vi "Init_Image_Dsts.vi"() -> (2 "Image Dsts Out":T2)   [LabVIEW 2011]
uses:
  <vilib>/vision/Image Controls.llb/IMAQ Image.ctl
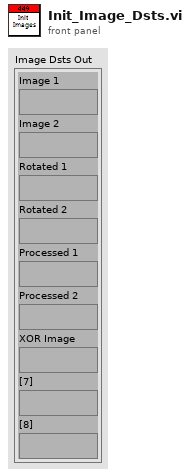
[diagram p1: front panel]
types:
  T1 = typedef "IMAQ Image.ctl" = refnum<image>
  T2 = cluster{"Image 1":T1, "Image 2":T1, "Rotated 1":T1, "Rotated 2":T1, "Processed 1":T1, "Processed 2":T1, "XOR Image":T1, "[7]":T1, "[8]":T1}
  T3 = typedef "Image Type" = u32
  T4 = cluster{"[0]":T1, "[1]":T1, "[2]":T1, "[3]":T1, "[4]":T1, "[5]":T1, "[6]":T1, "[7]":T1, "[8]":T1}
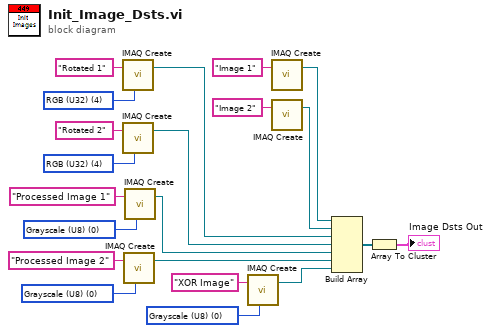
[diagram p0: block diagram]
diagram:
  w13 = T3 0 items=["Grayscale (U8)", "Grayscale (I16)", "Grayscale (SGL)", "Complex (CSG)", "RGB (U32)", "HSL (U32)", "RGB (U64)", "Grayscale (U16)"] ("Image Type")
  w15 = T3 0 items=["Grayscale (U8)", "Grayscale (I16)", "Grayscale (SGL)", "Complex (CSG)", "RGB (U32)", "HSL (U32)", "RGB (U64)", "Grayscale (U16)"] ("Image Type")
  w16 = T3 4 items=["Grayscale (U8)", "Grayscale (I16)", "Grayscale (SGL)", "Complex (CSG)", "RGB (U32)", "HSL (U32)", "RGB (U64)", "Grayscale (U16)"] ("Image Type")
  w18 = T3 4 items=["Grayscale (U8)", "Grayscale (I16)", "Grayscale (SGL)", "Complex (CSG)", "RGB (U32)", "HSL (U32)", "RGB (U64)", "Grayscale (U16)"] ("Image Type")
  w20 = T3 0 items=["Grayscale (U8)", "Grayscale (I16)", "Grayscale (SGL)", "Complex (CSG)", "RGB (U32)", "HSL (U32)", "RGB (U64)", "Grayscale (U16)"] ("Image Type")
  n1 = call "IMAQ Create"("Image Name"="Rotated 1", "Image Type"=w16) -> ("New Image"=w7:T1)  [unwired: 3 in, 1 out]
  n2 = call "IMAQ Create"("Image Name"="Rotated 2", "Image Type"=w18) -> ("New Image"=w6:T1)  [unwired: 3 in, 1 out]
  n3 = call "IMAQ Create"("Image Name"="Processed Image 2", "Image Type"=w15) -> ("New Image"=w4:T1)  [unwired: 3 in, 1 out]
  n4 = call "IMAQ Create"("Image Name"="Processed Image 1", "Image Type"=w20) -> ("New Image"=w5:T1)  [unwired: 3 in, 1 out]
  n5 = call "IMAQ Create"("Image Name"="XOR Image", "Image Type"=w13) -> ("New Image"=w3:T1)  [unwired: 3 in, 1 out]
  n6 = call "IMAQ Create"("Image Name"="Image 1") -> ("New Image"=w9:T1)  [unwired: 4 in, 1 out]
  n7 = call "IMAQ Create"("Image Name"="Image 2") -> ("New Image"=w8:T1)  [unwired: 4 in, 1 out]
  n8 = Build Array(w9, w8, w7, w6, w5, w4, w3) -> (w2:T1[])
  n9 = Array To Cluster(array=w2) -> (cluster=→"Image Dsts Out":T4)
